vi "Server Status.vi"(8 "entrée d'erreur (pas d'erreur)":errorcluster, 11 "Control en entrée":refnum<class "Control-Server.lvclass">) -> (0 "sortie d'erreur":errorcluster, 3 "Control en sortie":refnum<class "Control-Server.lvclass">)   [LabVIEW 2018, in "Control-Server.lvclass"]
uses:
  Classes/Control/Control-Server/Control-Server.lvclass
  C:/Users/Sergey Denisov/Documents/REPS/TRANCON/Classes/GeneralFunctionality/GeneralFunctionality.lvclass
  Clusters-def/Message types.ctl
  Clusters-def/Standard Command.ctl
  Clusters-def/SERVER-Commands.ctl
  Clusters-def/CONTROL-Reply-Status-client.ctl
  Clusters-def/DL-Reply-to-Connect-to-Client.ctl
  Clusters-def/DAQmx-Reply-Connect-client.ctl
  Clusters-def/OSc-Reply-Connect-client.ctl
  Clusters-def/Det-Reply-to-Connect-client.ctl
  Classes/Control/Control-Server/Control-Server.lvclass/Control-Server.ctl
  Classes/DAQmxTasks/DAQmxTaskContainer_General/DAQmxTaksContainer_General.lvclass
  Classes/Detector/Detector.lvclass
  Classes/Delay Line/DelayLine.lvclass
  Classes/Oscilloscope/Oscilloscope.lvclass
  Classes/Message/Message.lvclass
  Classes/Control/Control-Client/Control-Client.lvclass
  Classes/GeneralFunctionality/GeneralFunctionality.lvclass
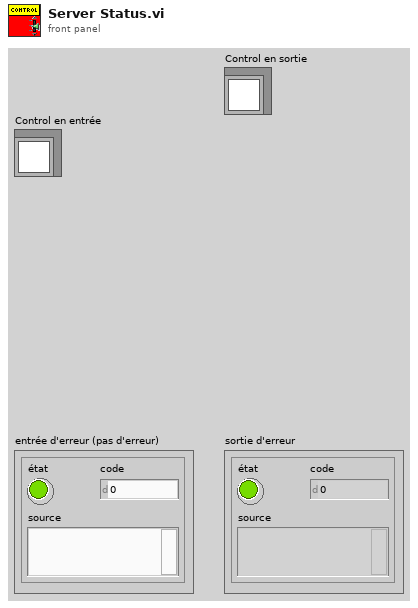
[diagram p1: front panel]
types:
  T1 = typedef "Control-Server.lvclass/SERVER-Commands.ctl" = string
  T2 = typedef "Standard Command.ctl" = cluster{"command":string, "data":variant}
  T3 = typedef "Message types.ctl" = string
  T4 = typedef "Oscilloscope.lvclass/OSc-Reply-Connect-client.ctl" = cluster{"on/off":bool, "WCM_state":bool, "error":errorcluster}
  T5 = typedef "Detector.lvclass/Det-Reply-to-Connect-client.ctl" = cluster{"on/off":bool, "calibration":dbl[], "error":errorcluster}
  T6 = typedef "DAQmxTaksContainer_General.lvclass/DAQmx-Reply-Connect-client.ctl" = cluster{"on/off":bool, "RelayKeyHeater/off":bool, "LaserShutter":bool, "AcceleratorShutter":bool, "Power":bool, "Faraday Cup Status":bool, "Pump Start_Stop":bool, "error":errorcluster}
  T7 = typedef "DelayLine.lvclass/DL-Reply-to-Connect-to-Client.ctl" = cluster{"on/off":bool, "position I":dbl, "position II":dbl, "Param":cluster{"Short":cluster{"min":dbl, "max":dbl, "real pos":dbl}, "Long":cluster{"min":dbl, "max":dbl, "real pos":dbl}}, "Cells_pos":dbl[], "error":errorcluster}
  T8 = typedef "Control-Client.lvclass/CONTROL-Reply-Status-client.ctl" = cluster{"DL reply to client":T7, "Det reply to client":cluster{"on/off":bool, "calibration":dbl[], "error out":errorcluster}, "DAQmx reply to client":T6, "OSc reply to CLIENT":T4}
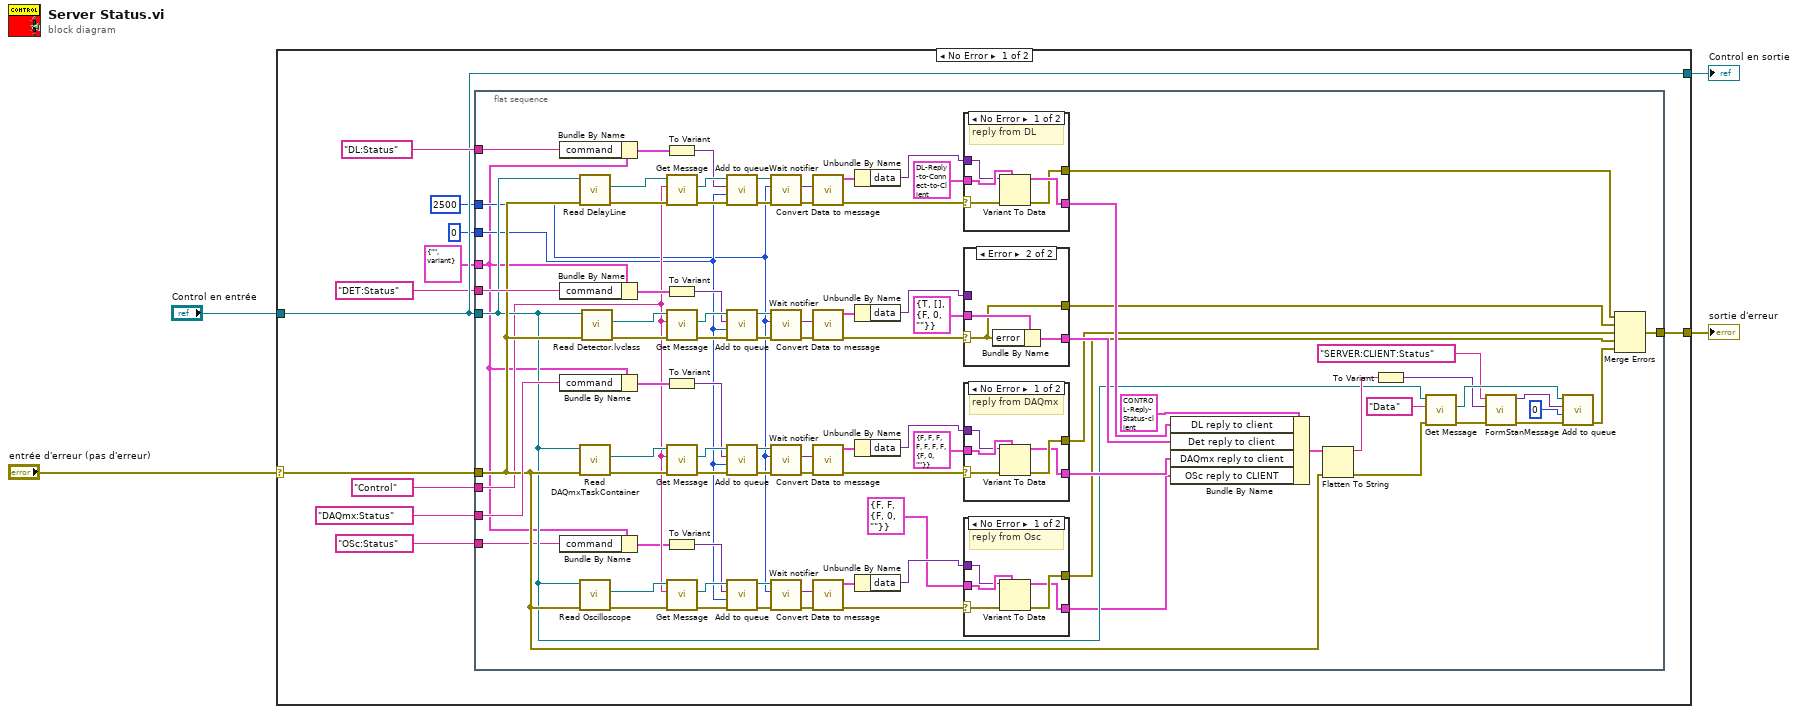
[diagram p0: block diagram]
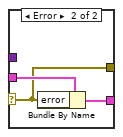
[diagram p2: hidden frame]
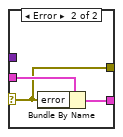
[diagram p3: hidden frame]
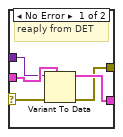
[diagram p4: hidden frame]
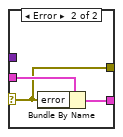
[diagram p5: hidden frame]
diagram:
  n1 = case shown="No Error" "entrée d'erreur (pas d'erreur)" {
    selector: "entrée d'erreur (pas d'erreur)" -> [w13 w136]
    tunnel: "Control en entrée" -> [w14 w137]
    tunnel: [w14 w137] -> w3
    tunnel: [w6 w136] -> w2
    frame No Error {
      n2 = flat-sequence {
        tunnel: T1 "DL:Status" ("Commands") -> [w99]
        tunnel: w14 -> [w38]
        tunnel: w13 -> [w39]
        tunnel: T3 "Control" ("Message type") -> [w29]
        tunnel: T1 "DET:Status" ("Commands") -> [w92]
        tunnel: T2 {"command"="", "data"=variant} ("input cluster") -> [w18]
        tunnel: T1 "DAQmx:Status" ("Commands") -> [w87]
        tunnel: 0 ("timeout in ms (-1)") -> [w27]
        tunnel: 2500 ("timeout in ms (-1)") -> [w26]
        tunnel: [w66] -> w6
        tunnel: T1 "OSc:Status" ("Commands") -> [w19]
        frame #0 {
          n3 = Bundle By Name(cluster=w18, "command"=w99) -> (w98:T2)
          n4 = Bundle By Name(cluster=w18, "command"=w92) -> (w89:T2)
          n5 = Bundle By Name(cluster=w18, "command"=w87) -> (w86:T2)
          n6 = Bundle By Name(cluster=w18, "command"=w19) -> (w17:T2)
          n7 = call "Read DelayLine.vi"("error in (no error)"=w39, "Control in"=w38) -> ("error out"=w100:errorcluster, "DelayLine.lvclass"=w101:refnum<class "DelayLine.lvclass">)  [unwired: 7 in, 1 out]
          n8 = call-dynamic "Read DAQmxTaskContainer.vi"("error in (no error)"=w39, "Control in"=w38) -> ("error out"=w96:errorcluster, "DAQmxTaksContainer_General.lvclass"=w95:refnum<class "DAQmxTaksContainer_General.lvclass">)  [unwired: 7 in, 1 out]
          n9 = call "Read Oscilloscope.vi"("error in (no error)"=w39, "Control-Server en entrée"=w38) -> ("error out"=w31:errorcluster, "Oscilloscope.lvclass"=w30:refnum<class "Oscilloscope.lvclass">)  [unwired: 7 in, 1 out]
          n10 = call "Read Detector.lvclass.vi"("error in (no error)"=w39, "Control in"=w38) -> ("error out"=w94:errorcluster, "Detector.lvclass"=w93:refnum<class "Detector.lvclass">)  [unwired: 7 in, 1 out]
          n11 = To Variant(anything=w98) -> (Variant=w97:variant)
          n12 = call "Get Message.vi"("error in (no error)"=w100, "Message type"=w29, "GeneralFunctionality en entrée"=w101) -> ("error out"=w102:errorcluster, "Message.lvclass"=w103:refnum<class "Message.lvclass">)  [unwired: 6 in, 1 out]
          n13 = To Variant(anything=w89) -> (Variant=w88:variant)
          n14 = call "Get Message.vi"("error in (no error)"=w94, "Message type"=w29, "GeneralFunctionality en entrée"=w93) -> ("error out"=w91:errorcluster, "Message.lvclass"=w90:refnum<class "Message.lvclass">)  [unwired: 6 in, 1 out]
          n15 = To Variant(anything=w86) -> (Variant=w77:variant)
          n16 = call "Get Message.vi"("error in (no error)"=w96, "Message type"=w29, "GeneralFunctionality en entrée"=w95) -> ("error out"=w84:errorcluster, "Message.lvclass"=w85:refnum<class "Message.lvclass">)  [unwired: 6 in, 1 out]
          n17 = To Variant(anything=w17) -> (Variant=w28:variant)
          n18 = call "Get Message.vi"("error in (no error)"=w31, "Message type"=w29, "GeneralFunctionality en entrée"=w30) -> ("error out"=w33:errorcluster, "Message.lvclass"=w32:refnum<class "Message.lvclass">)  [unwired: 6 in, 1 out]
          n19 = call "Add to queue.vi"("error in (no error)"=w102, "timeout in ms (-1)"=w27, "Data"=w97, "Message in"=w103) -> ("error out"=w83:errorcluster, "Message out"=w82:refnum<class "Message.lvclass">)  [unwired: 6 in]
          n20 = call "Add to queue.vi"("error in (no error)"=w91, "timeout in ms (-1)"=w27, "Data"=w88, "Message in"=w90) -> ("error out"=w81:errorcluster, "Message out"=w80:refnum<class "Message.lvclass">)  [unwired: 6 in]
          n21 = call "Add to queue.vi"("error in (no error)"=w84, "timeout in ms (-1)"=w27, "Data"=w77, "Message in"=w85) -> ("error out"=w79:errorcluster, "Message out"=w78:refnum<class "Message.lvclass">)  [unwired: 6 in]
          n22 = call "Add to queue.vi"("error in (no error)"=w33, "timeout in ms (-1)"=w27, "Data"=w28, "Message in"=w32) -> ("error out"=w34:errorcluster, "Message out"=w35:refnum<class "Message.lvclass">)  [unwired: 6 in]
          n23 = call "Wait notifier.vi"("error in (no error)"=w83, "timeout in ms (-1)"=w26, "Message en entrée"=w82) -> ("error out"=w44:errorcluster, "notification"=w43:variant)  [unwired: 6 in, 1 out]
          n24 = call "Wait notifier.vi"("error in (no error)"=w81, "timeout in ms (-1)"=w26, "Message en entrée"=w80) -> ("error out"=w49:errorcluster, "notification"=w48:variant)  [unwired: 6 in, 1 out]
          n25 = call "Wait notifier.vi"("error in (no error)"=w79, "timeout in ms (-1)"=w26, "Message en entrée"=w78) -> ("error out"=w54:errorcluster, "notification"=w52:variant)  [unwired: 6 in, 1 out]
          n26 = call "Wait notifier.vi"("error in (no error)"=w34, "timeout in ms (-1)"=w26, "Message en entrée"=w35) -> ("error out"=w36:errorcluster, "notification"=w37:variant)  [unwired: 6 in, 1 out]
          n27 = call "Convert Data to message.vi"("entrée d'erreur (pas d'erreur)"=w44, "data"=w43) -> ("sortie d'erreur"=w40:errorcluster, "output cluster message"=w42:T2)  [unwired: 8 in]
          n28 = call "Convert Data to message.vi"("entrée d'erreur (pas d'erreur)"=w49, "data"=w48) -> ("sortie d'erreur"=w45:errorcluster, "output cluster message"=w47:T2)  [unwired: 8 in]
          n29 = call "Convert Data to message.vi"("entrée d'erreur (pas d'erreur)"=w54, "data"=w52) -> ("sortie d'erreur"=w53:errorcluster, "output cluster message"=w51:T2)  [unwired: 8 in]
          n30 = call "Convert Data to message.vi"("entrée d'erreur (pas d'erreur)"=w36, "data"=w37) -> ("sortie d'erreur"=w23:errorcluster, "output cluster message"=w25:T2)  [unwired: 8 in]
          n31 = Unbundle By Name(w42) -> ("data"=w41:variant)
          n32 = Unbundle By Name(w47) -> ("data"=w46:variant)
          n33 = Unbundle By Name(w51) -> ("data"=w50:variant)
          n34 = Unbundle By Name(w25) -> ("data"=w24:variant)
          n35 = case shown="No Error" w40 {
            selector: w40 -> [w116 w117]
            tunnel: [w115 w118] -> w75
            tunnel: [w114 w117] -> w69
            tunnel: T7 {"on/off"=FALSE, "position I"=0.0, "position II"=0.0, "Param"={"Short"={"min"=0.0, "max"=0.0, "real pos"=0.0}, "Long"={"min"=0.0, "max"=0.0, "real pos"=0.0}}, "Cells_pos"=[], "error"={"status"=FALSE, "code"=0, "source"=""}} ("output cluster") -> [w113 w119]
            tunnel: w41 -> [w112 _]
            frame No Error {
              # "reply from DL"
              n36 = Variant To Data(error in=w116, type=w113, Variant=w112) -> (data=w115:T7, error out=w114:errorcluster)
            }
            frame Error {
              n37 = Bundle By Name(cluster=w119, "error"=w117) -> (w118:T7)
            }
          }
          n38 = case shown="Error" w45 {
            selector: w45 -> [w124 w125]
            tunnel: w46 -> [w120 _]
            tunnel: [w123 w126] -> w70
            tunnel: [w122 w125] -> w68
            tunnel: T5 {"on/off"=TRUE, "calibration"=[], "error"={"status"=FALSE, "code"=0, "source"=""}} ("Det replay to client") -> [w121 w127]
            frame No Error {
              # "reaply from DET"
              n39 = Variant To Data(error in=w124, type=w121, Variant=w120) -> (data=w123:T5, error out=w122:errorcluster)
            }
            frame Error {
              n40 = Bundle By Name(cluster=w127, "error"=w125) -> (w126:T5)
            }
          }
          n41 = case shown="No Error" w53 {
            selector: w53 -> [w132 w133]
            tunnel: w50 -> [w128 _]
            tunnel: [w131 w133] -> w67
            tunnel: [w130 w134] -> w74
            tunnel: T6 {"on/off"=FALSE, "RelayKeyHeater/off"=FALSE, "LaserShutter"=FALSE, "AcceleratorShutter"=FALSE, "Power"=FALSE, "Faraday Cup Status"=FALSE, "Pump Start_Stop"=FALSE, "error"={"status"=FALSE, "code"=0, "source"=""}} ("output cluster") -> [w129 w135]
            frame No Error {
              # "reply from DAQmx"
              n42 = Variant To Data(error in=w132, type=w129, Variant=w128) -> (data=w130:T6, error out=w131:errorcluster)
            }
            frame Error {
              n43 = Bundle By Name(cluster=w135, "error"=w133) -> (w134:T6)
            }
          }
          n44 = case shown="No Error" w23 {
            selector: w23 -> [w108 w109]
            tunnel: w24 -> [w104 _]
            tunnel: [w107 w109] -> w21
            tunnel: [w106 w110] -> w22
            tunnel: T4 {"on/off"=FALSE, "WCM_state"=FALSE, "error"={"status"=FALSE, "code"=0, "source"=""}} ("output cluster") -> [w105 w111]
            frame No Error {
              # "reply from Osc"
              n45 = Variant To Data(error in=w108, type=w105, Variant=w104) -> (data=w106:T4, error out=w107:errorcluster)
            }
            frame Error {
              n46 = Bundle By Name(cluster=w111, "error"=w109) -> (w110:T4)
            }
          }
          n47 = Bundle By Name(cluster=T8 {"DL reply to client"={"on/off"=FALSE, "position I"=0.0, "position II"=0.0, "Param"={"Short"={"min"=0.0, "max"=0.0, "real pos"=0.0}, "Long"={"min"=0.0, "max"=0.0, "real pos"=0.0}}, "Cells_pos"=[], "error"={"status"=FALSE, "code"=0, "source"=""}}, "Det reply to client"={"on/off"=TRUE, "calibration"=[], "error out"={"status"=FALSE, "code"=0, "source"=""}}, "DAQmx reply to client"={"on/off"=FALSE, "RelayKeyHeater/off"=FALSE, "LaserShutter"=FALSE, "AcceleratorShutter"=FALSE, "Power"=FALSE, "Faraday Cup Status"=FALSE, "Pump Start_Stop"=FALSE, "error"={"status"=FALSE, "code"=0, "source"=""}}, "OSc reply to CLIENT"={"on/off"=FALSE, "WCM_state"=FALSE, "error"={"status"=FALSE, "code"=0, "source"=""}}} ("output cluster"), "DL reply to client"=w75, "Det reply to client"=w70, "DAQmx reply to client"=w74, "OSc reply to CLIENT"=w22) -> (w65:T8)
          n48 = Flatten To String(anything=w65, error in (no error)=w39) -> (data string=w64:string, error out=w63:errorcluster)  [unwired: 2 in, 1 out]
          n49 = To Variant(anything=w64) -> (Variant=w58:variant)
          n50 = call "Get Message.vi"("error in (no error)"=w63, "Message type"=T3 "Data", "GeneralFunctionality en entrée"=w38) -> ("error out"=w56:errorcluster, "Message.lvclass"=w61:refnum<class "Message.lvclass">)  [unwired: 6 in, 1 out]
          n51 = call "FormStanMessage.vi"("error in"=w56, "data"=w58, "Command"=T1 "SERVER:CLIENT:Status" ("Commands")) -> ("error out"=w55:errorcluster, "message"=w57:variant)  [unwired: 7 in]
          n52 = call "Add to queue.vi"("error in (no error)"=w55, "timeout in ms (-1)"=0, "Data"=w57, "Message in"=w61) -> ("error out"=w20:errorcluster)  [unwired: 6 in, 1 out]
          n53 = Merge Errors(w69, w68, w67, w21, w20) -> (w66:errorcluster)
        }
      }
    }
    frame Error {
    }
  }
  "sortie d'erreur" <- w2
  "Control en sortie" <- w3
